vi "Current Elevator State.vi"(8 "error in (no error)":errorcluster, 10 "Elevator State":T1 {"Current Elevation" scale=0.0..100.0; "Current Travel Rate" scale=-1.0..1.0}, 11 "GTH-Down in":refnum<class "GTH-Down.lvclass">) -> (0 "error out":errorcluster, 3 "GTH-Down out":refnum<class "GTH-Down.lvclass">)   [LabVIEW 2014, in "Elevator.lvlib" / "EL-Go To Height.lvlib" / "GTH-Down.lvclass"]
uses:
  GTH-Down.lvclass
  Elevator Class/Elevator State.ctl
  <vilib>/ActorFramework/Actor/Actor.lvclass/Actor.ctl
  <vilib>/ActorFramework/Message Enqueuer/Message Enqueuer.lvclass/Message Enqueuer.ctl
  <vilib>/ActorFramework/Message Enqueuer/Init from Existing Queue.vi
  <vilib>/ActorFramework/Message Enqueuer/Enqueue.vi
  <vilib>/ActorFramework/Message Priority Queue/Priority Enqueue.vi
  <vilib>/ActorFramework/Message Enqueuer/Message Enqueuer.lvclass
  EL-Go To Height Messages/Go To Holding Msg/Go To Holding Msg.lvclass
  EL-Go To Height Class/EL-Go To Height.lvclass
  <vilib>/ActorFramework/Actor/Actor.lvclass
  Elevator Class/Elevator.lvclass
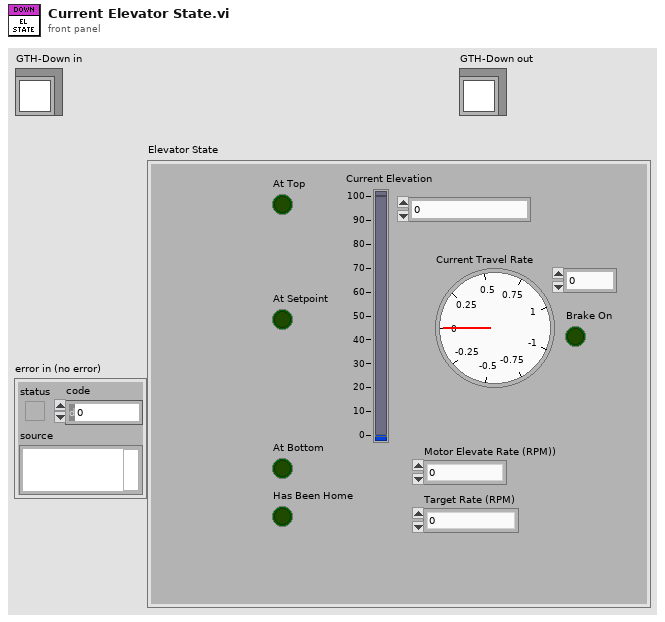
[diagram p1: front panel]
types:
  T1 = typedef "Elevator.lvlib/Elevator.lvclass/Elevator State.ctl" = cluster{"At Bottom":bool, "At Top":bool, "At Setpoint":bool, "Target Rate (RPM)":dbl, "Current Travel Rate":dbl, "Current Elevation":dbl, "Brake On":bool, "Motor Elevate Rate (RPM))":dbl, "Has Been Home":bool}
  T2 = typedef "Elevator.lvlib/EL-Go To Height.lvlib/EL-Go To Height.lvclass/Parameters.ctl" = cluster{"Target Height":dbl, "Elevator State Loop (ms)":u32, "Up Rate (Percentage)":dbl, "Down Rate (Percentage)":dbl}
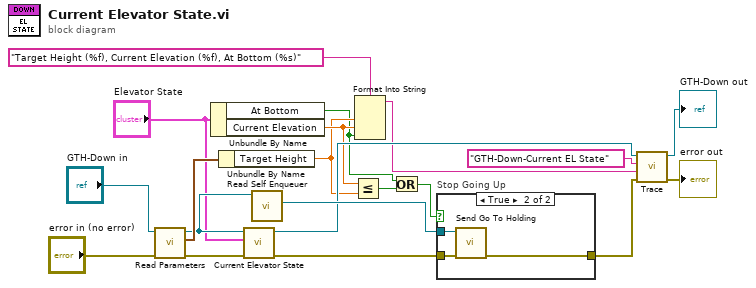
[diagram p0: block diagram]
diagram:
  n1 = call-dynamic "Read Parameters.vi"("error in (no error)"="error in (no error)", "EL-Go To Height in"="GTH-Down in") -> ("error out"=w18:errorcluster, "Parameters"=w17:T2, "EL-Go To Height out"=w12:refnum<class "GTH-Down.lvclass">)  [unwired: 7 in]
  n2 = Unbundle By Name("Elevator State") -> ("At Bottom"=w2:bool, "Current Elevation"=w5:dbl)
  n3 = Unbundle By Name(w17) -> ("Target Height"=w4:dbl)
  n4 = call-parent "Current Elevator State.vi"("error in (no error)"=w18, "Elevator State"="Elevator State", "EL-Go To Height in"=w12) -> ("error out"=w16:errorcluster, "EL-Go To Height out"=w10:refnum<class "GTH-Down.lvclass">)  [unwired: 7 in]
  n5 = call <vilib>:"Read Self Enqueuer.vi"("Actor"=w12) -> ("Self Enqueuer"=w11:refnum<class "Message Enqueuer.lvclass">)  [unwired: 10 in]
  n6 = Less Or Equal?(x=w5, y=w4) -> (x <= y?=w3:bool)
  n7 = Format Into String(format string="Target Height (%f), Current Elevation (%f), At Bottom (%s)", w4, w5, w2) -> (resulting string=w7:string)  [unwired: 2 in, 1 out]
  n8 = Or(x=w2, y=w3) -> (x .or. y?=w1:bool)
  n9 = case "Stop Going Up" shown="True" w1 {
    tunnel: w11 -> [_ w24]
    tunnel: w16 -> [w21 w23]
    tunnel: [w21 w22] -> w15
    frame False {
    }
    frame True {
      n10 = call "Send Go To Holding.vi"("error in (no error)"=w23, "Message Enqueuer"=w24) -> ("error out"=w22:errorcluster)  [unwired: 8 in, 1 out]
    }
  }
  n11 = call-dynamic "Trace.vi"("error in (no error)"=w15, "Command Message"=w7, "Command Action"="GTH-Down-Current EL State", "Command Actor in"=w10) -> ("error out"=→"error out":errorcluster, "Command Actor out"=→"GTH-Down out":refnum<class "GTH-Down.lvclass">)  [unwired: 6 in]
